vi "Calculo_Pressao.vi"(4 "X2":dbl, 5 "Valores":T1, 6 "Calibrador":bool, 7 "X":dbl) -> (0 "Pressao 2":dbl, 3 "Pressao":dbl)   [LabVIEW 2019]
panel:
  # "MAX"
  # "MIN"
  # "mmH2O"
  # "mmH2O"
  # "mm"
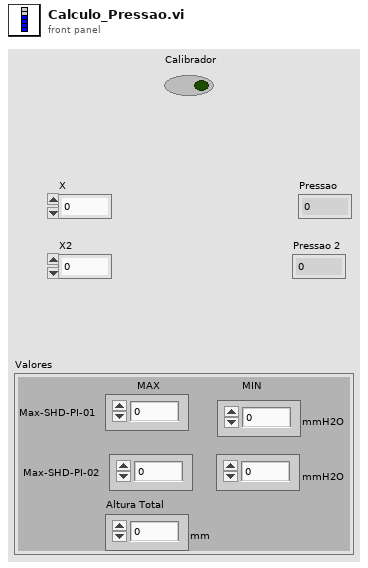
[diagram p1: front panel]
types:
  T1 = cluster{"Max-SHD-PI-01":i32, "Min-SIT-PI-FR1":i32, "Max-SHD-PI-02":i32, "Min-SIT-PI-FR2":i32, "Altura Total":i32}
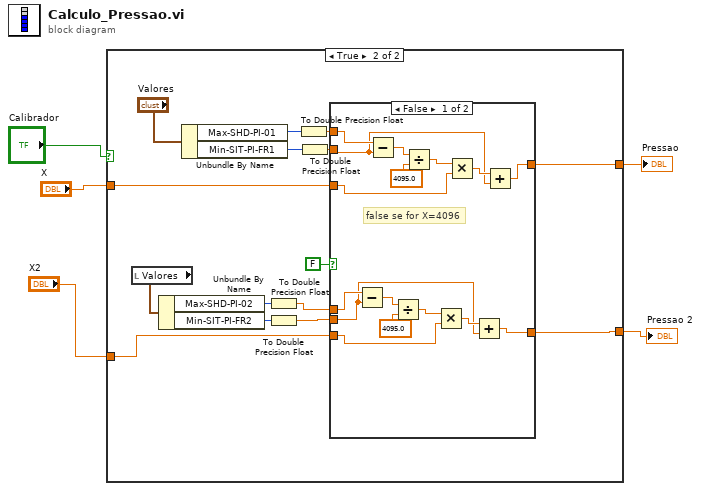
[diagram p0: block diagram]
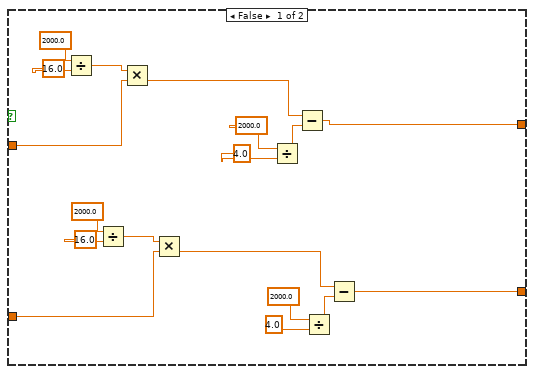
[diagram p2: hidden frame]
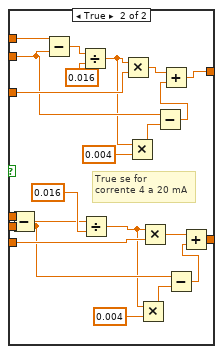
[diagram p3: hidden frame]
diagram:
  n1 = case shown="True" "Calibrador" {
    tunnel: "X" -> [w16 w31]
    tunnel: [w15 w29] -> w3
    tunnel: "X2" -> [w8 w28]
    tunnel: [w7 w27] -> w1
    frame False {
      n2 = Divide(x=2000.0, y=16.0) -> (x/y=w21:dbl)
      n3 = Divide(x=2000.0, y=16.0) -> (x/y=w13:dbl)
      n4 = Multiply(x=w21, y=w16) -> (x*y=w17:dbl)
      n5 = Multiply(x=w13, y=w8) -> (x*y=w9:dbl)
      n6 = Divide(x=2000.0, y=4.0) -> (x/y=w18:dbl)
      n7 = Subtract(x=w17, y=w18) -> (x-y=w15:dbl)
      n8 = Divide(x=2000.0, y=4.0) -> (x/y=w10:dbl)
      n9 = Subtract(x=w9, y=w10) -> (x-y=w7:dbl)
    }
    frame True {
      n10 = local read "Valores"() -> (w37:T1)
      n11 = Unbundle By Name(w37) -> ("Max-SHD-PI-02"=w33:i32, "Min-SIT-PI-FR2"=w34:i32)
      n12 = Unbundle By Name("Valores") -> ("Max-SHD-PI-01"=w35:i32, "Min-SIT-PI-FR1"=w30:i32)
      n13 = To Double Precision Float(number=w33) -> (double precision float=w32:dbl)
      n14 = To Double Precision Float(number=w34) -> (double precision float=w25:dbl)
      n15 = To Double Precision Float(number=w35) -> (double precision float=w36:dbl)
      n16 = To Double Precision Float(number=w30) -> (double precision float=w26:dbl)
      n17 = case shown="False" FALSE {
        tunnel: w36 -> [w51 w74]
        tunnel: w32 -> [w40 w73]
        tunnel: w31 -> [w50 w70]
        tunnel: [w47 w68] -> w29
        tunnel: w28 -> [w41 w67]
        tunnel: [w42 w65] -> w27
        tunnel: w26 -> [w48 w64]
        tunnel: w25 -> [w39 w56]
        frame False {
          # "false se for X=4096"
          n18 = Subtract(x=w40, y=w39) -> (x-y=w46:dbl)
          n19 = Subtract(x=w51, y=w48) -> (x-y=w54:dbl)
          n20 = Divide(x=w46, y=4095.0) -> (x/y=w43:dbl)
          n21 = Divide(x=w54, y=4095.0) -> (x/y=w49:dbl)
          n22 = Multiply(x=w43, y=w41) -> (x*y=w44:dbl)
          n23 = Multiply(x=w49, y=w50) -> (x*y=w52:dbl)
          n24 = Add(x=w44, y=w39) -> (x+y=w42:dbl)
          n25 = Add(x=w52, y=w48) -> (x+y=w47:dbl)
        }
        frame True {
          # "True se for \ncorrente 4 a 20 mA"
          n26 = Subtract(x=w73, y=w56) -> (x-y=w71:dbl)
          n27 = Subtract(x=w74, y=w64) -> (x-y=w76:dbl)
          n28 = Divide(x=w76, y=0.016) -> (x/y=w63:dbl)
          n29 = Divide(x=w71, y=0.016) -> (x/y=w55:dbl)
          n30 = Multiply(x=w63, y=w70) -> (x*y=w69:dbl)
          n31 = Multiply(x=w63, y=0.004) -> (x*y=w61:dbl)
          n32 = Multiply(x=w55, y=0.004) -> (x*y=w58:dbl)
          n33 = Multiply(x=w55, y=w67) -> (x*y=w66:dbl)
          n34 = Subtract(x=w64, y=w61) -> (x-y=w60:dbl)
          n35 = Add(x=w69, y=w60) -> (x+y=w68:dbl)
          n36 = Subtract(x=w56, y=w58) -> (x-y=w57:dbl)
          n37 = Add(x=w66, y=w57) -> (x+y=w65:dbl)
        }
      }
    }
  }
  "Pressao" <- w3
  "Pressao 2" <- w1
